vi "CGI Yield Calculate Data.vi"(11 "Yield Results":T1[](array[typedef])) -> (0 "# Sampled":i32, 1 "# Untested":i32, 2 "# Other":i32, 3 "# Pass":i32, 5 "Yield %":dbl)   [LabVIEW 2011]
uses:
  CGI Yield Results.ctl
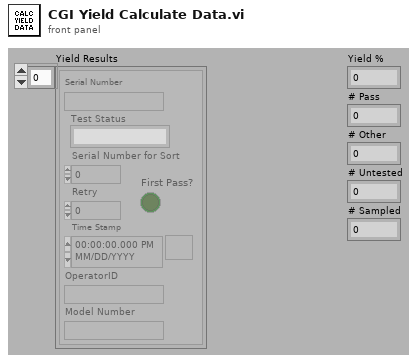
[diagram p1: front panel]
types:
  T1 = typedef "CGI Yield Results.ctl" = cluster{"Model Number":string, "Serial Number for Sort":i32, "Serial Number":string, "Test Status":string, "Time Stamp":timestamp, "OperatorID":string, "Retry":i32, "First Pass?":bool}
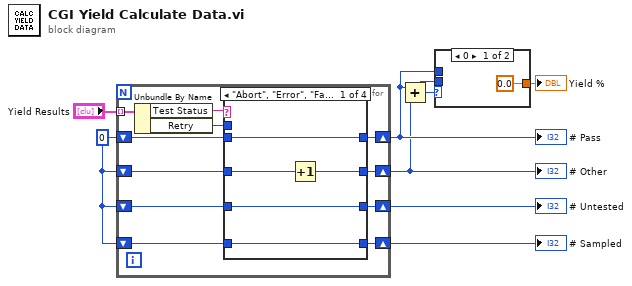
[diagram p0: block diagram]
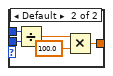
[diagram p2: hidden frame]
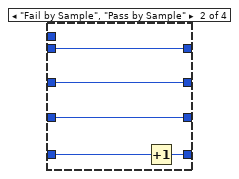
[diagram p3: hidden frame]
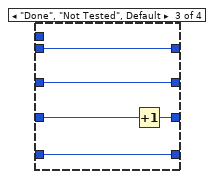
[diagram p4: hidden frame]
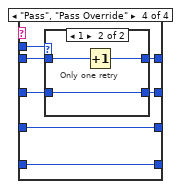
[diagram p5: hidden frame]
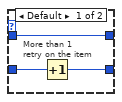
[diagram p6: hidden frame]
diagram:
  w7 = 0
  n1 = for {
    tunnel: "Yield Results" -> [w19] mode=indexing
    shift-right: [w13] -> w4
    shift-left: w7 -> [w17]
    shift-right: [w12] -> w3
    shift-left: w7 -> [w16]
    shift-right: [w11] -> w2
    shift-left: w7 -> [w15]
    shift-right: [w10] -> w1
    shift-left: w7 -> [w14]
    n2 = Unbundle By Name(w19) -> ("Test Status"=w18:string, "Retry"=w9:i32)
    n3 = case shown="\"Abort\", \"Error\", \"Fail\", \"Fail Override\"" w18 {
      tunnel: w17 -> [w24 w29 w34 w41]
      tunnel: w16 -> [w23 w28 w33 w36]
      tunnel: w15 -> [w22 w27 w32 w39]
      tunnel: w14 -> [w21 w26 w31 w38]
      tunnel: [w24 w29 w34 w40] -> w13
      tunnel: [w20 w28 w33 w35] -> w12
      tunnel: [w22 w27 w30 w39] -> w11
      tunnel: [w21 w25 w31 w38] -> w10
      tunnel: w9 -> [_ _ _ w37]
      frame "Abort", "Error", "Fail", "Fail Override" {
        n4 = Increment(x=w23) -> (x+1=w20:i32)
      }
      frame "Fail by Sample", "Pass by Sample" {
        n5 = Increment(x=w26) -> (x+1=w25:i32)
      }
      frame "Done", "Not Tested", Default {
        n6 = Increment(x=w32) -> (x+1=w30:i32)
      }
      frame "Pass", "Pass Override" {
        n7 = case shown="1" w37 {
          tunnel: w41 -> [w44 w47]
          tunnel: [w44 w46] -> w40
          tunnel: w36 -> [w43 w45]
          tunnel: [w42 w45] -> w35
          frame Default {
            # "More than 1\nretry on the item"
            n8 = Increment(x=w43) -> (x+1=w42:i32)
          }
          frame 1 {
            # "Only one retry"
            n9 = Increment(x=w47) -> (x+1=w46:i32)
          }
        }
      }
    }
  }
  "# Pass" <- w4
  "# Other" <- w3
  "# Untested" <- w2
  "# Sampled" <- w1
  n10 = Add(x=w4, y=w3) -> (x+y=w8:i32)
  n11 = case shown="0" w8 {
    tunnel: [0.0 w51] -> w5
    tunnel: w4 -> [_ w50]
    tunnel: w8 -> [_ w49]
    frame 0 {
    }
    frame Default {
      n12 = Divide(x=w50, y=w49) -> (x/y=w53:dbl)
      n13 = Multiply(x=w53, y=100.0) -> (x*y=w51:dbl)
    }
  }
  "Yield %" <- w5
